vi "dscDAConvertCode.vi"(6 "dscDASettings":T1 {"load_cal" items=["FALSE", "TRUE"]}, 8 "error in":errorcluster, 9 "voltage":dbl, 10 "channel":u8, 11 "board":i16) -> (0 "error out":errorcluster, 3 "boardOut":i16)   [LabVIEW 2011, in "Diamond Universal Driver.lvlib"]
doc: "VI converts a voltage to a code based on the cards current settings and outputs that code to the DA converter. The voltage will stay fixed on that channel until the voltage is updated."
uses:
  Diamond Universal Driver.lvlib
  Controls/dscDASettings.ctl
  Controls/dscPolarity.ctl
  Controls/dscBool.ctl
  Controls/error codes.ctl
  Instruments/WL OPC/Support/dlls/dscud.dll
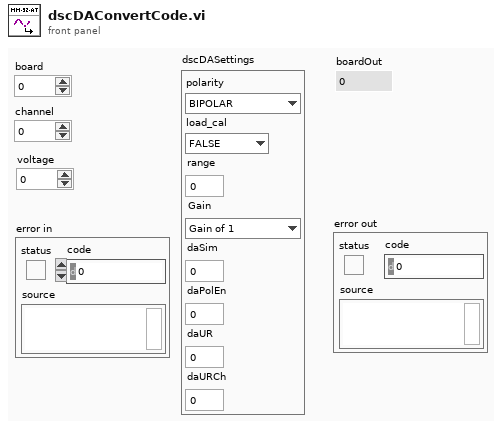
[diagram p1: front panel]
types:
  T1 = typedef "Diamond Universal Driver.lvlib/dscDASettings.ctl" = cluster{"polarity":T2, "load_cal":T3, "range":sgl, "Gain":enum16{"Gain of 1", "Gain of 2", "Gain of 4", "Gain of 8"}, "daSim":u8, "daPolEn":u8, "daUR":u8, "daURCh":u8}
  T2 = typedef "Diamond Universal Driver.lvlib/dscPolarity.ctl" = enum8{"BIPOLAR", "UNIPOLAR"}
  T3 = typedef "dscBool.ctl" = i32
  T4 = typedef "Diamond Universal Driver.lvlib/error codes.ctl" = enum8{"DE_NONE", "DE_HW_FAILURE", "DE_SW_FAILURE", "DE_HW_NOT_SUPPORTED", "DE_SW_NOT_SUPPORTED", "DE_INVALID_PARM", "DE_ALTERNATE_IN_PROGRESS", "DE_NONE_IN_PROGRESS", "DE_BUFFER_ROLLOVER", "DE_INVALID_ERROR_CODE", "DE_ALREADY_PAUSED", "DE_OVERFLOW", "DE_INVALID_FUNC", "DE_DSCUDH_INVALID", "DE_INVALID_BOARD", "DE_BOARD_LIMIT_REACHED", "DE_BOARD_BUSY", "DE_INVALID_WINDRVR_HANDLE", "DE_INVALID_WINDRVR_VERSION", "DE_BAD_WINDRVR_BOARD_INIT", "DE_OPERATION_TIMED_OUT", "DE_INVALID_WINDRVR_KP", "DE_THREAD_FAILURE"}
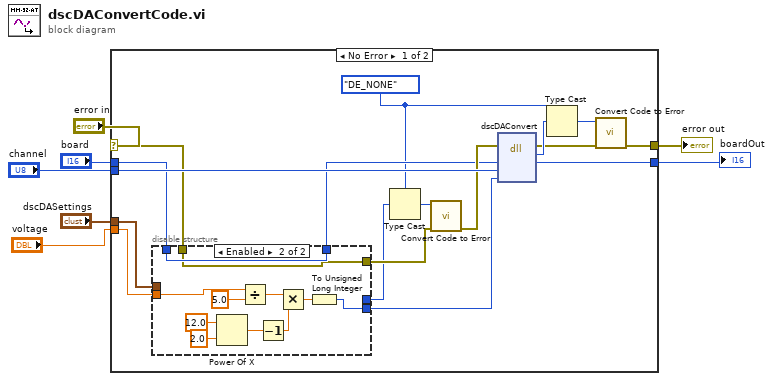
[diagram p0: block diagram]
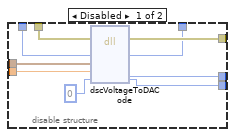
[diagram p2: hidden frame]
diagram:
  n1 = case shown="No Error" "error in" {
    selector: "error in" -> [w15 w46]
    tunnel: "board" -> [w13 w45]
    tunnel: [w21 w45] -> w5
    tunnel: [w20 w46] -> w4
    tunnel: "channel" -> [w19 _]
    tunnel: "dscDASettings" -> [w18 _]
    tunnel: "voltage" -> [w10 _]
    frame No Error {
      w11 = error_codes."DE_NONE" ("error codes")
      n2 = disable-structure shown="Enabled" {
        disable-tunnel: w18 -> [w33 _]
        disable-tunnel: [w31 _] -> w9
        disable-tunnel: [w30 w35] -> w16
        disable-tunnel: w15 -> [w29 w35]
        disable-tunnel: w13 -> [w28 w36]
        disable-tunnel: [w27 w36] -> w12
        disable-tunnel: w10 -> [w26 w37]
        disable-tunnel: [w25 w34] -> w8
        frame Disabled {
          n3 = dll-call lib="C:/Users/mrichardson/Documents/Web Based Version Control SW/Instruments/WL OPC/Support/dlls/dscud.dll" fn="dscVoltageToDACode"(error in=w29, "board"=w28, "dasettings"=w33, "voltage"=w26, "dacode"=u32 0) -> (error out=w30:errorcluster, "error"=w31:u8, "board"=w27:i16, "dacode"=w25:u32)  [unwired: 4 in, 1 out]
        }
        frame Enabled {
          n4 = Power Of X(1:2.0 ("x"), 2:12.0 ("y")) -> (0:w42:dbl)
          n5 = Divide(x=w37, y=5.0) -> (x/y=w39:dbl)
          n6 = Decrement(x=w42) -> (x-1=w43:dbl)
          n7 = Multiply(x=w39, y=w43) -> (x*y=w44:dbl)
          n8 = To Unsigned Long Integer(number=w44) -> (unsigned 32bit integer=w34:u32)
        }
      }
      n9 = Type Cast(type=w11, x=w9) -> (*(type *) &x=w17:T4)
      n10 = call "Convert Code to Error.vi"("error in"=w16, "error codes"=w17) -> ("error out"=w14:errorcluster)  [unwired: 9 in]
      n11 = dll-call lib="C:/Users/mrichardson/Documents/Web Based Version Control SW/Instruments/WL OPC/Support/dlls/dscud.dll" fn="dscDAConvert"(error in=w14, "board"=w12, "channel"=w19, "output_code"=w8) -> (error out=w22:errorcluster, "error"=w23:u8, "board"=w21:i16)  [unwired: 4 in, 1 out]
      n12 = Type Cast(type=w11, x=w23) -> (*(type *) &x=w24:T4)
      n13 = call "Convert Code to Error.vi"("error in"=w22, "error codes"=w24) -> ("error out"=w20:errorcluster)  [unwired: 9 in]
    }
    frame Error {
    }
  }
  "boardOut" <- w5
  "error out" <- w4
